vi "Find Leaks.vi"(4 "error in":errorcluster, 6 "String File":path, 7 "Secrets Configuration":path) -> (0 "error out":errorcluster, 2 "String File Dup":path, 3 "Leaks":T1[](array[typedef]))   [LabVIEW 2025]
doc: "This VI searches the <b>String File</b> for secrets defined in the <b>Secrets Configuration</b> XML file. If any secret is found, this VI will produce the custom error -8000: \"Code Contains Secrets\".\n\nThe <b>Leaks</b> Output contains an array of all Leaks (i.e. Secrets with Value) found."
uses:
  Type Definitions/Leak--cluster.ctl
  Type Definitions/Secret--cluster.ctl
  <vilib>/regexp/Match Regular Expression.xnode
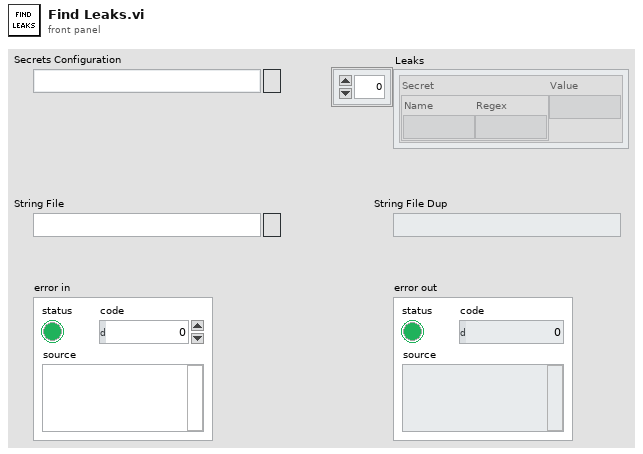
[diagram p1: front panel]
types:
  T1 = typedef "Leak--cluster.ctl" = cluster{"Secret":T2, "Value":string}
  T2 = typedef "Secret--cluster.ctl" = cluster{"Name":string, "Regex":string}
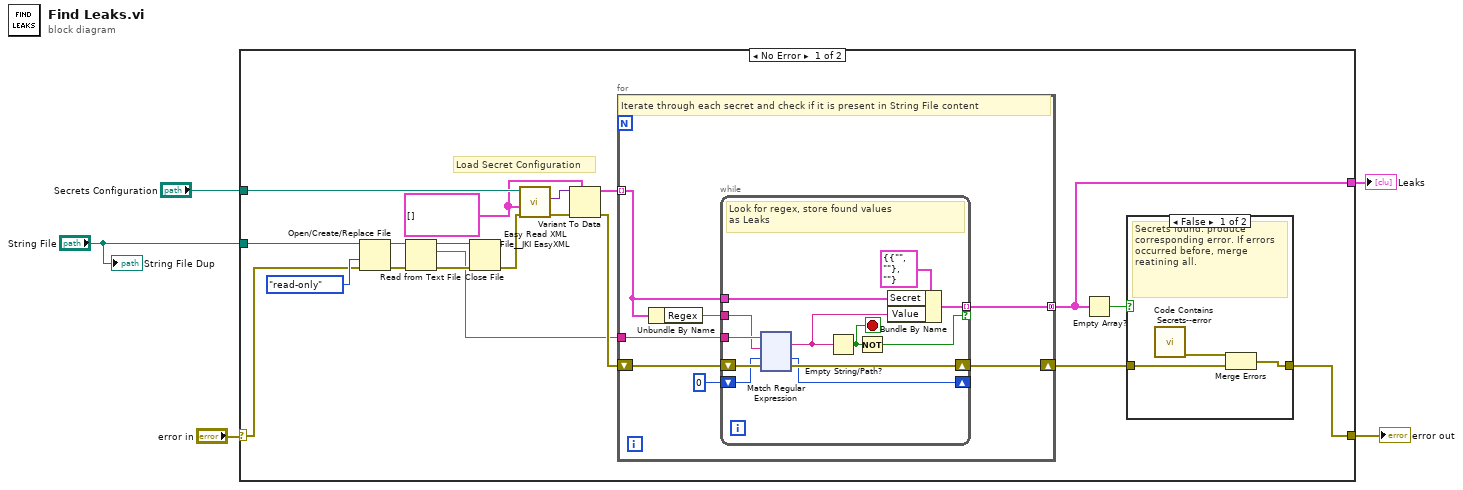
[diagram p0: block diagram]
diagram:
  n1 = case shown="No Error" "error in" {
    selector: "error in" -> [w10 w165]
    tunnel: "String File" -> [w20 _]
    tunnel: "Secrets Configuration" -> [w18 _]
    tunnel: [w9 w165] -> w2
    tunnel: [w6 _] -> w1
    frame No Error {
      w15 = T2[] [] ("Array")
      # "Load Secret Configuration"
      n2 = Open/Create/Replace File(file path (use dialog)=w20, error in=w10, access (0:read/write)=enum16{"read/write", "read-only", "write-only"}."read-only") -> (refnum out=w24:refnum<file>, error out=w23:errorcluster)  [unwired: 3 in, 1 out]
      n3 = Read from Text File(file (use dialog)=w24, error in=w23) -> (refnum out=w21:refnum<file>, text=w11:string, error out=w22:errorcluster)  [unwired: 2 in, 1 out]
      n4 = Close File(refnum=w21, error in=w22) -> (error out=w13:errorcluster)  [unwired: 1 out]
      n5 = call <vilib>:"Easy Read XML File__JKI EasyXML.vi"("error in (no error)"=w13, "LabVIEW Data (Type)"=w15, "XML File Path"=w18) -> ("error out"=w17:errorcluster, "LabVIEW Data"=w16:variant)  [unwired: 6 in, 1 out]
      n6 = Variant To Data(error in=w17, type=w15, Variant=w16) -> (data=w14:T2[], error out=w12:errorcluster)
      n7 = for {
        tunnel: w14 -> [w30] mode=indexing
        tunnel: w11 -> [w35]
        shift-right: [w32] -> w8
        shift-left: w12 -> [w33]
        tunnel: [w29] -> w6 mode=concatenating
        # "Iterate through each secret and check if it is present in String File content"
        n8 = Unbundle By Name(w30) -> ("Regex"=w34:string)
        n9 = while {
          tunnel: w35 -> [w47]
          tunnel: w34 -> [w46]
          shift-right: [w44] -> w32
          shift-left: w33 -> [w45]
          shift-right: [w42] -> _
          shift-left: 0 -> [w43]
          tunnel: [w38] -> w29 mode=indexing if=w41
          tunnel: w30 -> [w39]
          stop <- w36 stop-if-true
          # "Look for regex, store found values\nas Leaks"
          n10 = xnode "Match Regular Expression"("input string"=w47, "regular expression"=w46, "offset (0)"=w43, "error in"=w45) -> ("whole match"=w37:string, "offset past match"=w42:i32, "error out"=w44:errorcluster)  [unwired: 2 in, 2 out]
          n11 = Empty String/Path?(string/path=w37) -> (empty?=w36:bool)
          n12 = Not(x=w36) -> (.not. x?=w41:bool)
          n13 = Bundle By Name(cluster=T1 {"Secret"={"Name"="", "Regex"=""}, "Value"=""} ("Leak"), "Secret"=w39, "Value"=w37) -> (w38:T1)
        }
      }
      n14 = Empty Array?(array=w6) -> (empty?=w7:bool)
      n15 = case shown="False" w7 {
        tunnel: w8 -> [w26 w28]
        tunnel: [w27 w28] -> w9
        frame False {
          # "Secrets found: produce corresponding error. If errors occurred before, merge reatining all."
          n16 = call "Code Contains Secrets--error.vi"() -> ("error out"=w25:errorcluster)  [unwired: 7 in]
          n17 = Merge Errors(w25, w26) -> (w27:errorcluster)
        }
        frame True {
          # "No secrets found: pass error"
        }
      }
    }
    frame Error {
    }
  }
  "error out" <- w2
  "Leaks" <- w1
  "String File Dup" <- "String File"
